vi "hAdres2014.vi"(4 "error in":errorcluster, 5 "Kanal#":u8, 6 "AdressMode":enum16{"select", "oben", "unten", "keinen"}(ring), 7 "FPGA VI Reference In":refnum<k20>) -> (0 "error out":errorcluster, 3 "FPGA VI Reference Out":refnum<k20>)   [LabVIEW 2014]
doc: "Wählt je nach Auswahl alle oberen bzw unteren oder einen einzelnen Kanal aus."
uses:
  <vilib>/Utility/error.llb/Error Cluster From Error Code.vi
  <vilib>/rvi/errors/niLvFpgaAdjustHostInterfaceError.vi
  <vilib>/rvi/interface/nirviReadWriteControl/nirviReadWriteControl.xnode
  FPGA Bitfiles/W7XBolo2017_FPGATarget_FlorianDefault.lvbitx
  f_main_2014.vi
  NiFpgaLv.dll
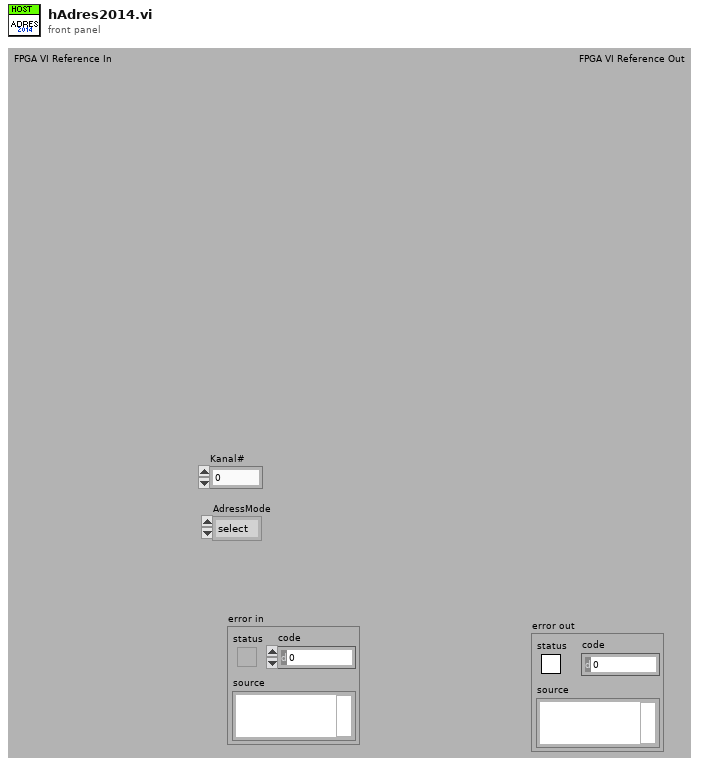
[diagram p1: front panel]
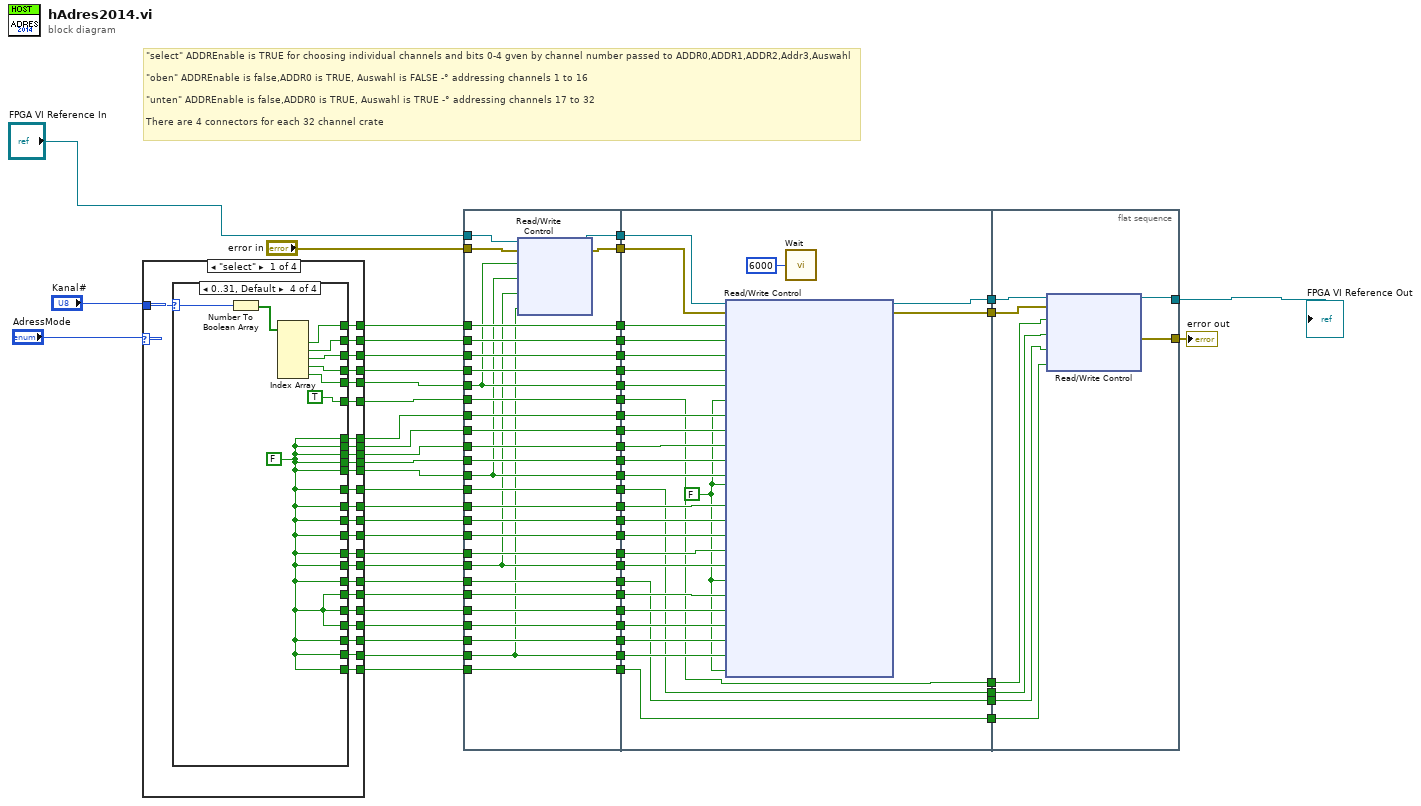
[diagram p0: block diagram]
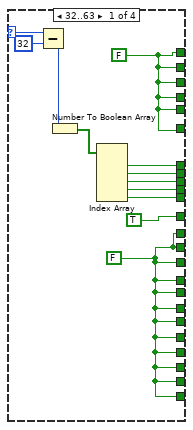
[diagram p2: hidden frame]
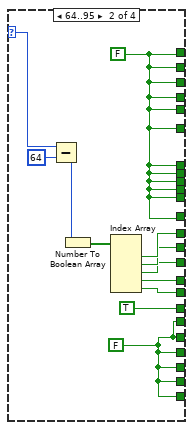
[diagram p3: hidden frame]
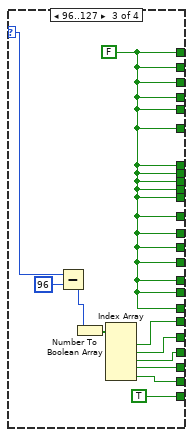
[diagram p4: hidden frame]
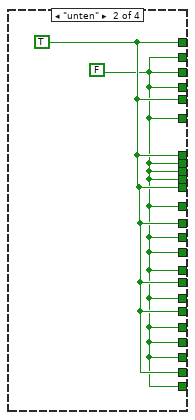
[diagram p5: hidden frame]
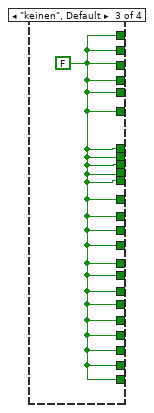
[diagram p6: hidden frame]
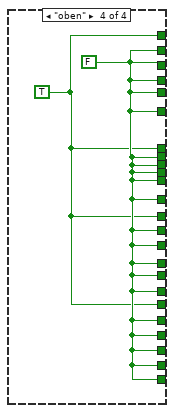
[diagram p7: hidden frame]
diagram:
  # "\"select\" ADDREnable is TRUE for choosing individual channels and bits 0-4 gven by channel number passed to ADDR0,ADDR1,ADDR2,Addr3,Auswahl\n\n\"oben\" ADDREnable is false,ADDR0 is TRUE, Auswahl is FALSE -° addressing channels 1 to 16\n\n\"unten\" ADDREnable is false,ADDR0 is TRUE, Auswahl is TRUE -° addressing channels 17 to 32\n\nThere are 4 connectors for each 32 channel crate"
  n1 = case shown="\"select\"" "AdressMode" {
    tunnel: "Kanal#" -> [w81 _ _ _]
    tunnel: [w86 w132 w134 w136] -> w61
    tunnel: [w85 w133 w134 w135] -> w60
    tunnel: [w84 w132 w134 w136] -> w59
    tunnel: [w87 w132 w134 w136] -> w58
    tunnel: [w83 w132 w134 w136] -> w57
    tunnel: [w82 w133 w134 w136] -> w56
    tunnel: [w80 w133 w134 w136] -> w49
    tunnel: [w79 w132 w134 w136] -> w50
    tunnel: [w78 w132 w134 w136] -> w51
    tunnel: [w77 w132 w134 w136] -> w52
    tunnel: [w76 w133 w134 w135] -> w53
    tunnel: [w75 w132 w134 w136] -> w48
    tunnel: [w74 w133 w134 w135] -> w42
    tunnel: [w73 w132 w134 w136] -> w43
    tunnel: [w72 w132 w134 w136] -> w44
    tunnel: [w71 w132 w134 w136] -> w45
    tunnel: [w70 w133 w134 w136] -> w46
    tunnel: [w69 w132 w134 w136] -> w47
    tunnel: [w68 w133 w134 w135] -> w38
    tunnel: [w67 w132 w134 w136] -> w37
    tunnel: [w63 w132 w134 w136] -> w36
    tunnel: [w66 w132 w134 w136] -> w39
    tunnel: [w65 w133 w134 w136] -> w40
    tunnel: [w64 w132 w134 w136] -> w41
    frame "select" {
      n2 = case shown="0..31, Default" w81 {
        selector: w81 -> [w98 w108 w119 w124]
        tunnel: [w89 w101 w112 w130] -> w87
        tunnel: [w89 w101 w112 TRUE] -> w86
        tunnel: [w89 w101 w112 w128] -> w85
        tunnel: [w89 w101 w112 w127] -> w84
        tunnel: [w89 w101 w112 w126] -> w83
        tunnel: [w89 w101 w112 w125] -> w82
        tunnel: [w95 w101 w112 w123] -> w80
        tunnel: [w94 w101 w112 w123] -> w79
        tunnel: [w93 w101 w112 w123] -> w78
        tunnel: [w92 w101 w112 w123] -> w77
        tunnel: [w91 w101 w112 w123] -> w76
        tunnel: [TRUE w101 w112 w123] -> w75
        tunnel: [w88 w107 w112 w123] -> w74
        tunnel: [w88 w106 w112 w123] -> w73
        tunnel: [w88 w105 w112 w123] -> w72
        tunnel: [w88 w104 w112 w123] -> w71
        tunnel: [w88 w103 w112 w123] -> w70
        tunnel: [w88 TRUE w112 w123] -> w69
        tunnel: [w88 w100 w118 w123] -> w68
        tunnel: [w88 w100 w117 w123] -> w67
        tunnel: [w88 w100 w115 w123] -> w66
        tunnel: [w88 w100 w114 w123] -> w65
        tunnel: [w88 w100 TRUE w123] -> w64
        tunnel: [w88 w100 w116 w123] -> w63
        frame 32..63 {
          w88 = FALSE
          w89 = FALSE
          n3 = Subtract(x=w98, y=u8 32) -> (x-y=w96:u8)
          n4 = Number To Boolean Array(number=w96) -> (Boolean array=w99:bool[])
          n5 = Index Array(array=w99) -> (element #1=w91:bool, element #2=w92:bool, element #3=w93:bool, element #4=w94:bool, element #5=w95:bool)  [unwired: 5 in]
        }
        frame 64..95 {
          w100 = FALSE
          w101 = FALSE
          n6 = Subtract(x=w108, y=u8 64) -> (x-y=w109:u8)
          n7 = Number To Boolean Array(number=w109) -> (Boolean array=w111:bool[])
          n8 = Index Array(array=w111) -> (element #1=w107:bool, element #2=w106:bool, element #3=w105:bool, element #4=w104:bool, element #5=w103:bool)  [unwired: 5 in]
        }
        frame 96..127 {
          w112 = FALSE
          n9 = Subtract(x=w119, y=u8 96) -> (x-y=w120:u8)
          n10 = Number To Boolean Array(number=w120) -> (Boolean array=w122:bool[])
          n11 = Index Array(array=w122) -> (element #1=w118:bool, element #2=w117:bool, element #3=w116:bool, element #4=w115:bool, element #5=w114:bool)  [unwired: 5 in]
        }
        frame 0..31, Default {
          w123 = FALSE
          n12 = Number To Boolean Array(number=w124) -> (Boolean array=w131:bool[])
          n13 = Index Array(array=w131) -> (element #1=w128:bool, element #2=w127:bool, element #3=w130:bool, element #4=w126:bool, element #5=w125:bool)  [unwired: 5 in]
        }
      }
    }
    frame "unten" {
      w132 = FALSE
      w133 = TRUE
    }
    frame "keinen", Default {
      w134 = FALSE
    }
    frame "oben" {
      w136 = FALSE
      w135 = TRUE
    }
  }
  n14 = flat-sequence {
    tunnel: w36 -> [w144]
    tunnel: w37 -> [w145]
    tunnel: w38 -> [w146]
    tunnel: w39 -> [w147]
    tunnel: w40 -> [w137]
    tunnel: w41 -> [w148]
    tunnel: w42 -> [w149]
    tunnel: w43 -> [w150]
    tunnel: w44 -> [w151]
    tunnel: w45 -> [w152]
    tunnel: w46 -> [w138]
    tunnel: w47 -> [w153]
    tunnel: w48 -> [w154]
    tunnel: w49 -> [w139]
    tunnel: w50 -> [w155]
    tunnel: w51 -> [w156]
    tunnel: w52 -> [w157]
    tunnel: w53 -> [w158]
    tunnel: "FPGA VI Reference In" -> [w159]
    tunnel: w56 -> [w140]
    tunnel: w57 -> [w160]
    tunnel: w58 -> [w161]
    tunnel: w59 -> [w162]
    tunnel: w60 -> [w163]
    tunnel: w61 -> [w164]
    tunnel: "error in" -> [w142]
    tunnel: [w141] -> w35
    tunnel: [w164] -> w34
    tunnel: [w163] -> w33
    tunnel: [w162] -> w32
    tunnel: [w161] -> w31
    tunnel: [w160] -> w30
    tunnel: [w140] -> w29
    tunnel: [w143] -> w28
    tunnel: [w158] -> w27
    tunnel: [w157] -> w26
    tunnel: [w156] -> w25
    tunnel: [w155] -> w24
    tunnel: [w139] -> w23
    tunnel: [w154] -> w22
    tunnel: [w153] -> w21
    tunnel: [w138] -> w20
    tunnel: [w152] -> w19
    tunnel: [w151] -> w18
    tunnel: [w150] -> w17
    tunnel: [w149] -> w16
    tunnel: [w148] -> w15
    tunnel: [w137] -> w14
    tunnel: [w147] -> w13
    tunnel: [w146] -> w12
    tunnel: [w145] -> w11
    tunnel: [w144] -> w10
    tunnel: w35 -> [w194]
    tunnel: w34 -> [w165]
    tunnel: w33 -> [w193]
    tunnel: w32 -> [w192]
    tunnel: w31 -> [w191]
    tunnel: w30 -> [w190]
    tunnel: w29 -> [w189]
    tunnel: w28 -> [w186]
    tunnel: w27 -> [w184]
    tunnel: w26 -> [w183]
    tunnel: w25 -> [w182]
    tunnel: w24 -> [w181]
    tunnel: w23 -> [w180]
    tunnel: w22 -> [w166]
    tunnel: w21 -> [w167]
    tunnel: w20 -> [w179]
    tunnel: w19 -> [w178]
    tunnel: w18 -> [w177]
    tunnel: w17 -> [w176]
    tunnel: w16 -> [w175]
    tunnel: w15 -> [w168]
    tunnel: w14 -> [w170]
    tunnel: w13 -> [w174]
    tunnel: w12 -> [w173]
    tunnel: w11 -> [w172]
    tunnel: w10 -> [w171]
    tunnel: [w188] -> w9
    tunnel: [w187] -> w8
    tunnel: [w168] -> w6
    tunnel: [w167] -> w5
    tunnel: [w166] -> w4
    tunnel: [w165] -> w3
    tunnel: [w199] -> w2
    tunnel: w9 -> [w202]
    tunnel: w8 -> [w201]
    tunnel: [w200] -> w7
    tunnel: w6 -> [w198]
    tunnel: w5 -> [w197]
    tunnel: w4 -> [w196]
    tunnel: w3 -> [w195]
    frame #0 {
      n15 = xnode "Read/Write Control"("FPGA VI Reference In"=w159, "error in"=w142, "C0Auswahl"=w140, "C1Auswahl"=w139, "C2Auswahl"=w138, "C3Auswahl"=w137) -> ("FPGA VI Reference Out"=w143:refnum<k20>, "error out"=w141:errorcluster)
    }
    frame #1 {
      w169 = FALSE
      n16 = xnode "Read/Write Control"("FPGA VI Reference In"=w186, "error in"=w194, "C0ADDR0"=w193, "C0ADDR1"=w192, "C0ADDR2"=w191, "C0ADDR3"=w190, "C0Auswahl"=w189, "C0ADDREnable"=w169, "C1ADDR0"=w184, "C1ADDR1"=w183, "C1ADDR2"=w182, "C1ADDR3"=w181, "C1Auswahl"=w180, "C1ADDREnable"=w169, "C2ADDR0"=w175, "C2ADDR1"=w176, "C2ADDR2"=w177, "C2ADDR3"=w178, "C2Auswahl"=w179, "C2ADDREnable"=w169, "C3ADDR0"=w173, "C3ADDR1"=w172, "C3ADDR2"=w171, "C3ADDR3"=w174, "C3Auswahl"=w170, "C3ADDREnable"=w169) -> ("FPGA VI Reference Out"=w188:refnum<k20>, "error out"=w187:errorcluster)
      n17 = call "Wait"("Count(uSec)"=u32 6000) -> ()  [unwired: 1 out]
    }
    frame #2 {
      n18 = xnode "Read/Write Control"("FPGA VI Reference In"=w202, "error in"=w201, "C0ADDREnable"=w195, "C1ADDREnable"=w196, "C2ADDREnable"=w197, "C3ADDREnable"=w198) -> ("FPGA VI Reference Out"=w199:refnum<k20>, "error out"=w200:errorcluster)
    }
  }
  "error out" <- w7
  "FPGA VI Reference Out" <- w2
